vi "Sprawdzenie czy robot znajduje się w zadanym promieniu od wskazanego punktu.vi"(6 "Odległość od startu [m] 2":cluster{"X [m]":dbl, "Y [m]":dbl}, 9 "Wybór punktu":u16, 10 "Lista współrzędnych":string[][](array[string]), 11 "zad. promien odlegl.":dbl) -> (3 "Boolean":bool)   [LabVIEW 2012]
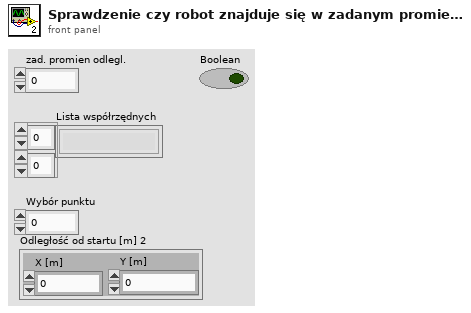
[diagram p1: front panel]
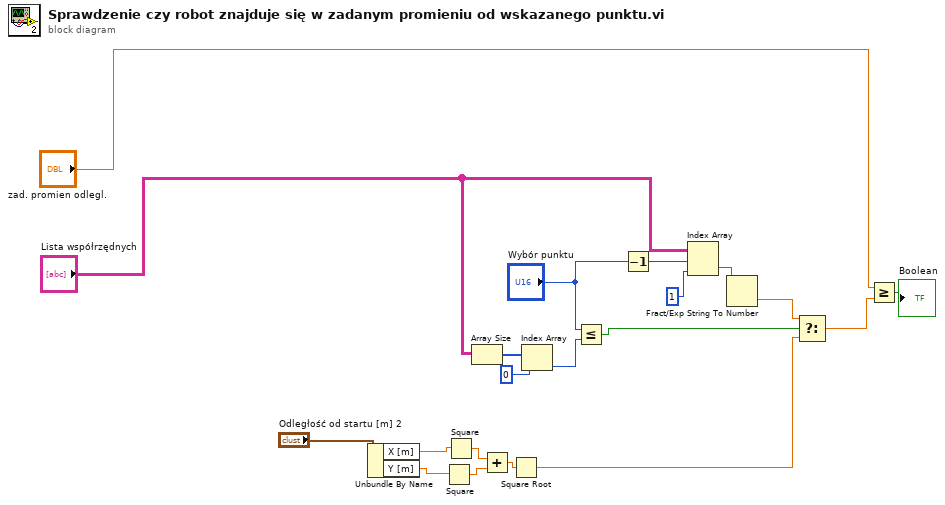
[diagram p0: block diagram]
diagram:
  n1 = Unbundle By Name("Odległość od startu [m] 2") -> ("X [m]"=w6:dbl, "Y [m]"=w5:dbl)
  n2 = Square(x=w5) -> (x^2=w4:dbl)
  n3 = Square(x=w6) -> (x^2=w3:dbl)
  n4 = Array Size(array="Lista współrzędnych") -> (size(s)=w13:i32[])
  n5 = Add(x=w3, y=w4) -> (x+y=w2:dbl)
  n6 = Square Root(x=w2) -> (sqrt(x)=w1:dbl)
  n7 = Index Array(array=w13, index=0) -> (element=w12:i32)
  n8 = Less Or Equal?(x="Wybór punktu", y=w12) -> (x <= y?=w10:bool)
  n9 = Decrement(x="Wybór punktu") -> (x-1=w20:u16)
  n10 = Index Array(array="Lista współrzędnych", index (row)=w20, index (col)=1 ("disabled index (col)")) -> (element=w18:string)
  n11 = Fract/Exp String To Number(string=w18) -> (number=w9:dbl)  [unwired: 3 in, 1 out]
  n12 = Select(t=w9, s=w10, f=w1) -> (s? t:f=w8:dbl)
  n13 = Greater Or Equal?(x="zad. promien odlegl.", y=w8) -> (x >= y?=→"Boolean":bool)
